vi "CheckBit.vi"(1 "Match bit":u8=4, 2 "MM2000 Address (Hexadecimal)":u32=832 format="%.0x") -> (0 "Match?":bool)   [LabVIEW 2022 SP3]
panel:
  out "HEX Out":u8 format="%.0b"
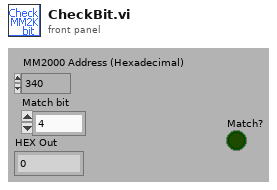
[diagram p1: front panel]
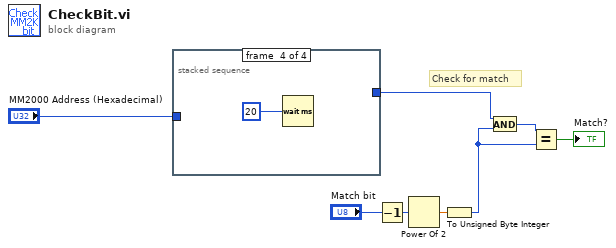
[diagram p0: block diagram]
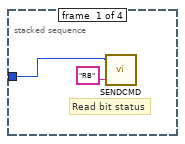
[diagram p2: hidden frame]
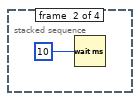
[diagram p3: hidden frame]
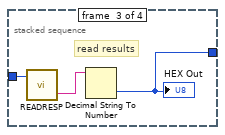
[diagram p4: hidden frame]
diagram:
  # "Check for match"
  n1 = stacked-sequence {
    tunnel: "MM2000 Address (Hexadecimal)" -> [w9 _ w14 _]
    tunnel: [_ _ w12 _] -> w6
    frame #0 {
      # "Read bit status"
      n2 = call "SENDCMD.VI"("MM2000 Command (ASCII String)"="RB", "MM2000 Address (Hexadecimal)"=w9) -> ()  [unwired: 1 in, 1 out]
    }
    frame #1 {
      n3 = Wait (ms)(milliseconds to wait=10) -> ()  [unwired: 1 out]
    }
    frame #2 {
      # "read results"
      n4 = call "READRESP.VI"("MM2000 Address (Hexadecimal)"=w14) -> ("MM2000 Response (ASCII String)"=w13:string)
      n5 = Decimal String To Number(string=w13) -> (number=w12:i32)  [unwired: 1 in, 2 out]
      "HEX Out" <- w12
    }
    frame #3 {
      n6 = Wait (ms)(milliseconds to wait=20) -> ()  [unwired: 1 out]
    }
  }
  n7 = Decrement(x="Match bit") -> (x-1=w2:u8)
  n8 = Power Of 2(x=w2) -> (2^x=w3:dbl)
  n9 = To Unsigned Byte Integer(number=w3) -> (unsigned 8bit integer=w1:u8)
  n10 = And(x=w6, y=w1) -> (x .and. y?=w5:i32)
  n11 = Equal?(x=w5, y=w1) -> (x = y?=→"Match?":bool)
